vi "Dynamic Form.vi"(8 "error in (no error)":errorcluster, 9 "form outfile":path, 11 "instrument handle":refnum<k15>) -> (0 "error out":errorcluster, 1 "final current (A)":dbl, 2 "final resistance (ohm)":dbl format="%#_6p", 3 "instrument handle out":refnum<k15>, 4 "formed?":bool, 5 "WL voltage (V)":dbl, 7 "BL voltage (V)":dbl)   [LabVIEW 2018]
uses:
  Globals.vi
  <instrlib>/niDigital/niDigital.llb/niDigital Burst Pattern (Burst Only).vi
  <vilib>/Utility/file.llb/Write Delimited Spreadsheet (DBL).vi
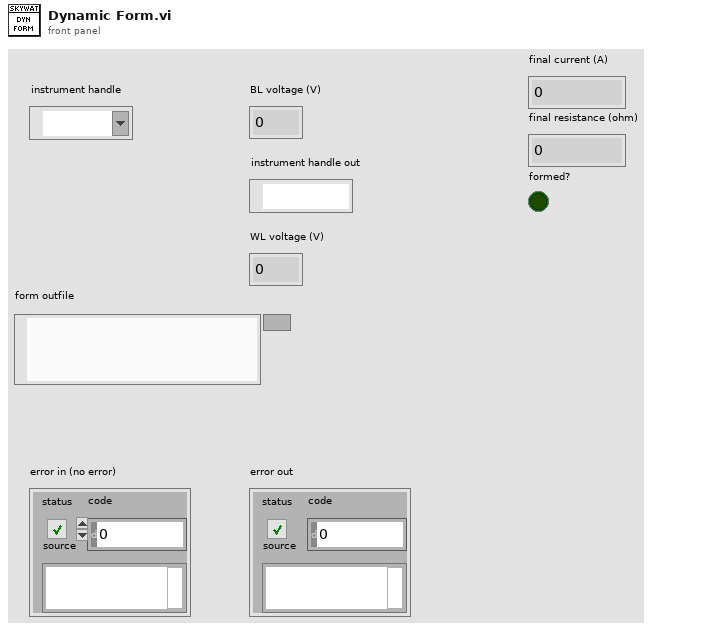
[diagram p1: front panel]
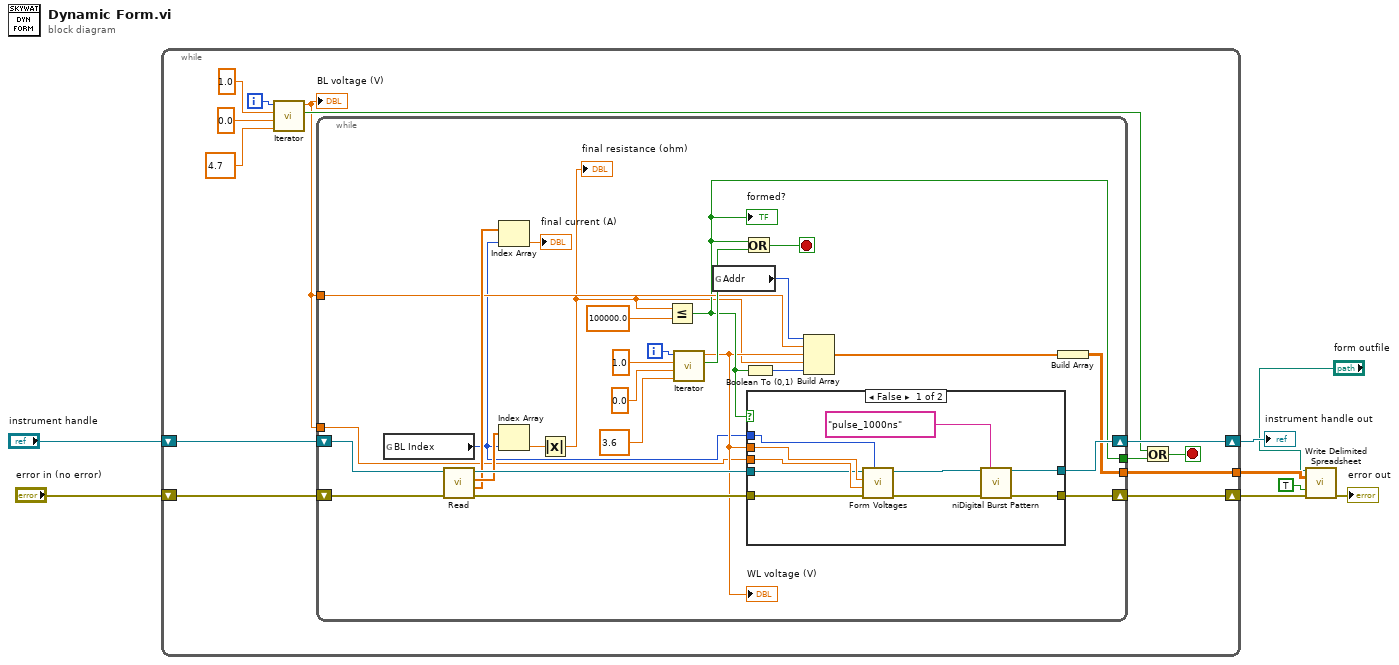
[diagram p0: block diagram]
diagram:
  n1 = while {
    shift-right: [w17] -> w8
    shift-left: "instrument handle" -> [w14]
    shift-right: [w16] -> w3
    shift-left: "error in (no error)" -> [w13]
    tunnel: [w9] -> w7
    i -> [w18]
    stop <- w19 stop-if-true
    n2 = call "Iterator.vi"("Final Value"=4.7 ("y"), "Initial Value"=0.0 ("y"), "Step"=1.0 ("x"), "i"=w18) -> ("End Loop"=w15:bool, "Current Value"=w10:dbl)  [unwired: 6 in]
    "BL voltage (V)" <- w10
    n3 = while {
      shift-right: [w47] -> w17
      shift-left: w14 -> [w43]
      shift-right: [w26] -> w16
      shift-left: w13 -> [w46]
      tunnel: w10 -> [w31]
      tunnel: [w30] -> w11
      tunnel: w10 -> [w28]
      tunnel: [w27] -> w9
      i -> [w42]
      stop <- w48 stop-if-true
      n4 = global read "Globals.vi" "BL Index"() -> (w22:i32)
      n5 = call "Read.vi"("error in (no error)"=w46, "instrument handle"=w43) -> ("error out"=w45:errorcluster, "currents (A)"=w35:dbl[], "resistances (ohm)"=w37:dbl[], "instrument handle out"=w44:refnum<k15>)  [unwired: 6 in]
      n6 = Index Array(array=w35, index=w22) -> (element=→"final current (A)":dbl)
      n7 = Index Array(array=w37, index=w22) -> (element=w24:dbl)
      n8 = Absolute Value(x=w24) -> (abs(x)=w23:dbl)
      "final resistance (ohm)" <- w23
      n9 = Less Or Equal?(x=w23, y=100000.0 ("target resistance (ohm)")) -> (x <= y?=w30:bool)
      "formed?" <- w30
      n10 = call "Iterator.vi"("Final Value"=3.6 ("y"), "Initial Value"=0.0 ("y"), "Step"=1.0 ("x"), "i"=w42) -> ("End Loop"=w38:bool, "Current Value"=w29:dbl)  [unwired: 6 in]
      "WL voltage (V)" <- w29
      n11 = global read "Globals.vi" "Addr"() -> (w25:i32)
      n12 = Or(x=w30, y=w38) -> (x .or. y?=w48:bool)
      n13 = Boolean To (0,1)(Boolean=w30) -> (0, 1=w34:i16)
      n14 = case shown="False" w30 {
        tunnel: [w58 w59] -> w26
        tunnel: [w57 w60] -> w47
        tunnel: w45 -> [w50 w59]
        tunnel: w44 -> [w49 w60]
        tunnel: w29 -> [w55 _]
        tunnel: w28 -> [w54 _]
        tunnel: w22 -> [w51 _]
        frame False {
          n15 = call "Form Voltages.vi"("index"=w51, "error in (no error)"=w50, "BL Voltage (V)"=w54, "WL Voltage (V)"=w55, "IVI Refnum in"=w49) -> ("error out"=w53:errorcluster, "IVI Refnum out"=w52:refnum<k15>)  [unwired: 5 in]
          n16 = call-poly <instrlib>:"niDigital Burst Pattern.vi"("instrument handle"=w52, "start label"="pulse_1000ns", "error in"=w53) -> ("instrument handle out"=w57:refnum<k15>, "error out"=w58:errorcluster)  [unwired: 11 in]
        }
        frame True {
        }
      }
      n17 = Build Array(w25, w31, w29, w23, w34) -> (w33:dbl[])
      n18 = Build Array(w33) -> (w27:dbl[][])
    }
    n19 = Or(x=w15, y=w11) -> (x .or. y?=w19:bool)
  }
  "instrument handle out" <- w8
  n20 = call-poly <vilib>:"Write Delimited Spreadsheet.vi"("file path (dialog if empty)"="form outfile", "2D data"=w7, "append to file? (new file:F)"=TRUE, "error in (no error)"=w3) -> ("error out"=→"error out":errorcluster)  [unwired: 10 in, 1 out]
